vi "Day 03 Part 2.vi"(11 "Input":string) -> (3 "Output":u32)   [LabVIEW 2021]
uses:
  <userlib>/_OpenG.lib/array/array.llb/Search 1D Array (I16)__ogtk.vi
  <userlib>/_OpenG.lib/array/array.llb/Delete Elements from 2D Array (U8)__ogtk.vi
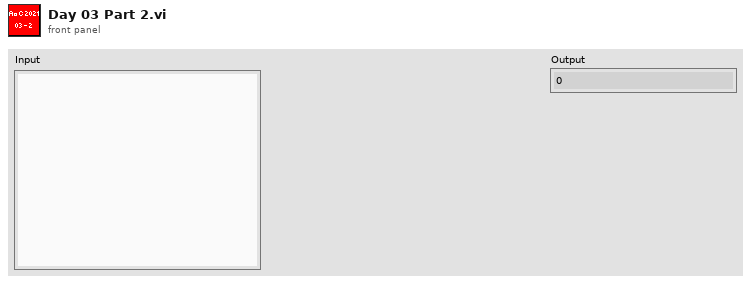
[diagram p1: front panel]
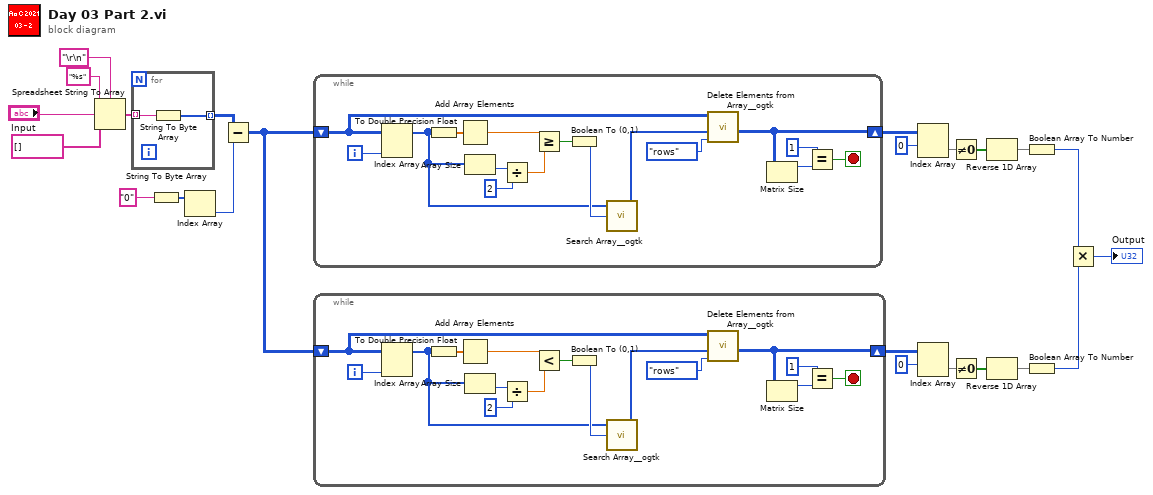
[diagram p0: block diagram]
diagram:
  n1 = Spreadsheet String To Array(delimiter (Tab)="\r\n", format string="%s", spreadsheet string="Input", array type (2D Dbl)=string[] []) -> (array=w20:string[])
  n2 = for {
    tunnel: w20 -> [w25] mode=indexing
    tunnel: [w24] -> w16 mode=indexing
    n3 = String To Byte Array(string=w25) -> (unsigned byte array=w24:u8[])
  }
  n4 = String To Byte Array(string="0" ("delimiter (Tab)")) -> (unsigned byte array=w18:u8[])
  n5 = Index Array(array=w18) -> (element=w17:u8)  [unwired: 1 in]
  n6 = Subtract(x=w16, y=w17) -> (x-y=w3:u8[][])
  n7 = while {
    shift-right: [w26] -> w13
    shift-left: w3 -> [w32]
    i -> [w33]
    stop <- w29 stop-if-true
    n8 = Index Array(array=w32, index (col)=w33) -> (element=w34:u8[])  [unwired: 1 in]
    n9 = To Double Precision Float(number=w34) -> (double precision float=w37:dbl[])
    n10 = Add Array Elements(numeric array=w37) -> (sum=w39:dbl)
    n11 = Array Size(array=w34) -> (size(s)=w41:i32)
    n12 = Divide(x=w41, y=2) -> (x/y=w38:dbl)
    n13 = Greater Or Equal?(x=w39, y=w38) -> (x >= y?=w36:bool)
    n14 = Boolean To (0,1)(Boolean=w36) -> (0, 1=w35:i16)
    n15 = call-poly <userlib>:"Search Array__ogtk.vi"("Array"=w34, "Element Data"=w35) -> ("Indices of Elements"=w31:i32[])  [unwired: 7 in]
    n16 = call-poly <userlib>:"Delete Elements from Array__ogtk.vi"("delete (rows or columns)"=enum16{"rows", "columns"}."rows", "indices"=w31, "array"=w32) -> ("deleted elements"=w26:u8[][])  [unwired: 7 in, 1 out]
    n17 = Matrix Size(0:w26) -> (1:w30:i32)  [unwired: 1 out]
    n18 = Equal?(x=1, y=w30) -> (x = y?=w29:bool)
  }
  n19 = while {
    shift-right: [w42] -> w5
    shift-left: w3 -> [w48]
    i -> [w49]
    stop <- w45 stop-if-true
    n20 = Index Array(array=w48, index (col)=w49) -> (element=w50:u8[])  [unwired: 1 in]
    n21 = To Double Precision Float(number=w50) -> (double precision float=w53:dbl[])
    n22 = Add Array Elements(numeric array=w53) -> (sum=w55:dbl)
    n23 = Array Size(array=w50) -> (size(s)=w57:i32)
    n24 = Divide(x=w57, y=2) -> (x/y=w54:dbl)
    n25 = Less?(x=w55, y=w54) -> (x < y?=w52:bool)
    n26 = Boolean To (0,1)(Boolean=w52) -> (0, 1=w51:i16)
    n27 = call-poly <userlib>:"Search Array__ogtk.vi"("Array"=w50, "Element Data"=w51) -> ("Indices of Elements"=w47:i32[])  [unwired: 7 in]
    n28 = call-poly <userlib>:"Delete Elements from Array__ogtk.vi"("delete (rows or columns)"=enum16{"rows", "columns"}."rows", "indices"=w47, "array"=w48) -> ("deleted elements"=w42:u8[][])  [unwired: 7 in, 1 out]
    n29 = Matrix Size(0:w42) -> (1:w46:i32)  [unwired: 1 out]
    n30 = Equal?(x=1, y=w46) -> (x = y?=w45:bool)
  }
  n31 = Index Array(array=w13, index (row)=0) -> (element=w11:u8[])  [unwired: 1 in]
  n32 = Index Array(array=w5, index (row)=0) -> (element=w7:u8[])  [unwired: 1 in]
  n33 = Not Equal To 0?(x=w11) -> (x != 0?=w10:bool[])
  n34 = Not Equal To 0?(x=w7) -> (x != 0?=w8:bool[])
  n35 = Reverse 1D Array(array=w10) -> (reversed array=w15:bool[])
  n36 = Reverse 1D Array(array=w8) -> (reversed array=w4:bool[])
  n37 = Boolean Array To Number(Boolean array=w15) -> (number=w1:u32)
  n38 = Boolean Array To Number(Boolean array=w4) -> (number=w2:u32)
  n39 = Multiply(x=w1, y=w2) -> (x*y=→"Output":u32)
